vi "Check_one_device_is_busy.vi"(0 "DEVICE_SN":string, 2 "USB_DEV_json":string) -> (14 "USB_DEV_Json":string, 16 "Device?":bool)   [LabVIEW 2015]
uses:
  Share Data/uPower_kit.ctl
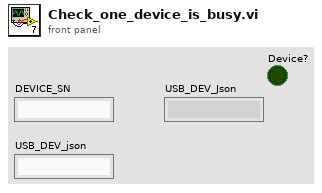
[diagram p1: front panel]
types:
  T1 = typedef "uPower_kit.ctl" = cluster{"DEV":string, "BUSY":bool, "VBAT":dbl, "OUTPUT":bool, "LAST_RESULT":dbl, "DURATION":u16, "TRIGGER":bool, "RANGE":string, "Vsource":dbl}
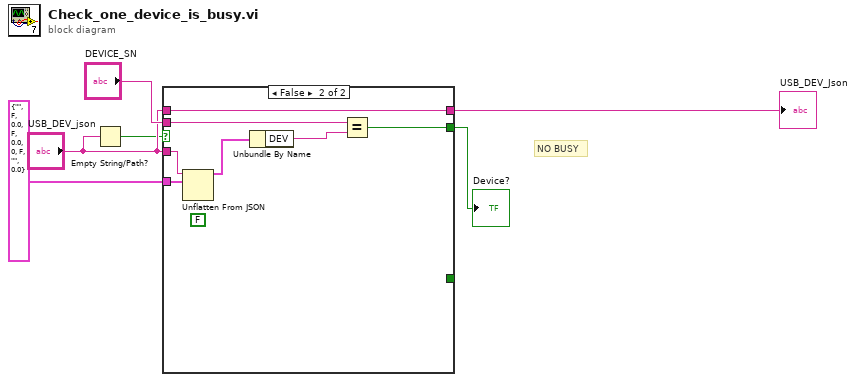
[diagram p0: block diagram]
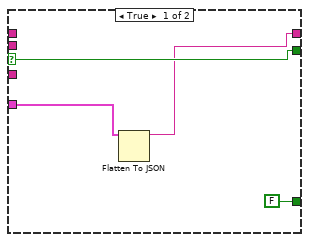
[diagram p2: hidden frame]
diagram:
  # "NO BUSY"
  n1 = Empty String/Path?(string/path="USB_DEV_json") -> (empty?=w3:bool)
  n2 = case shown="False" w3 {
    selector: w3 -> [w10 _]
    tunnel: "USB_DEV_json" -> [_ w17]
    tunnel: T1 {"DEV"="", "BUSY"=FALSE, "VBAT"=0.0, "OUTPUT"=FALSE, "LAST_RESULT"=0.0, "DURATION"=0, "TRIGGER"=FALSE, "RANGE"="", "Vsource"=0.0} ("DEV_BUSY") -> [w8 w16]
    tunnel: "DEVICE_SN" -> [_ w13]
    tunnel: [w10 w11] -> w4
    tunnel: [w7 w12] -> w1
    tunnel: "USB_DEV_json" -> [_ w12]
    tunnel: [FALSE ("BUSY") _] -> _
    frame True {
      n3 = Flatten To JSON(anything=w8) -> (JSON string=w7:string)  [unwired: 2 in, 1 out]
    }
    frame False {
      (unwired) FALSE ("f")
      n4 = Unflatten From JSON(JSON string=w17, type and defaults=w16) -> (value=w15:T1)  [unwired: 5 in, 1 out]
      n5 = Unbundle By Name(w15) -> ("DEV"=w14:string)
      n6 = Equal?(x=w13, y=w14) -> (x = y?=w11:bool)
    }
  }
  "USB_DEV_Json" <- w1
  "Device?" <- w4
